vi "ArmControl.vi"   [LabVIEW 2012]
uses:
  Robot Global Data.vi
  State_Machine_Enum.ctl
  <vilib>/Rock Robotics/WPI/Relay/WPI_RelayValue.ctl
types:
  T1 = typedef "State_Machine_Enum.ctl" = enum16{"Idle", "Start", "Do", "Stop", "Init"}
  T2 = typedef "WPI_RelayValue.ctl" = enum16{"Off", "On", "Forward", "Reverse"}
  T3 = typedef "LoopDisable.ctl" = cluster{"Climb.vi":bool, "LauncherAngle.vi":bool, "Launcher.vi":bool, "ArmControl.vi":bool, "WinchMotor.vi":bool, "ReadDriveEncoder.vi":bool}
  T4 = typedef "WPI_RelayDevRef.ctl" = cluster{"DevStatus":errorcluster, "Relay Channel":T5, "Digital Module":T6, "Relay Direction":T7}
  T5 = typedef "FPGA_DIORelayChannel.ctl" = enum8{"Relay 1", "Relay 2", "Relay 3", "Relay 4", "Relay 5", "Relay 6", "Relay 7", "Relay 8", "Invalid"}
  T6 = typedef "FPGA_TypedefDigitalModule.ctl" = enum16{"Digital Module 1", "Digital Module 2"}
  T7 = typedef "WPI_RelayDirection.ctl" = enum16{"Both directions", "Forward only", "Reverse only"}
  T8 = typedef "WPI_DigitalInputDevRef.ctl" = cluster{"DevStatus":errorcluster, "DIO Channel":T9, "Digital Module":T6}
  T9 = typedef "FPGA_DIOChannel.ctl" = enum8{"DIO 1", "DIO 2", "DIO 3", "DIO 4", "DIO 5", "DIO 6", "DIO 7", "DIO 8", "DIO 9", "DIO 10", "DIO 11", "DIO 12", "DIO 13", "DIO 14", "Invalid"}
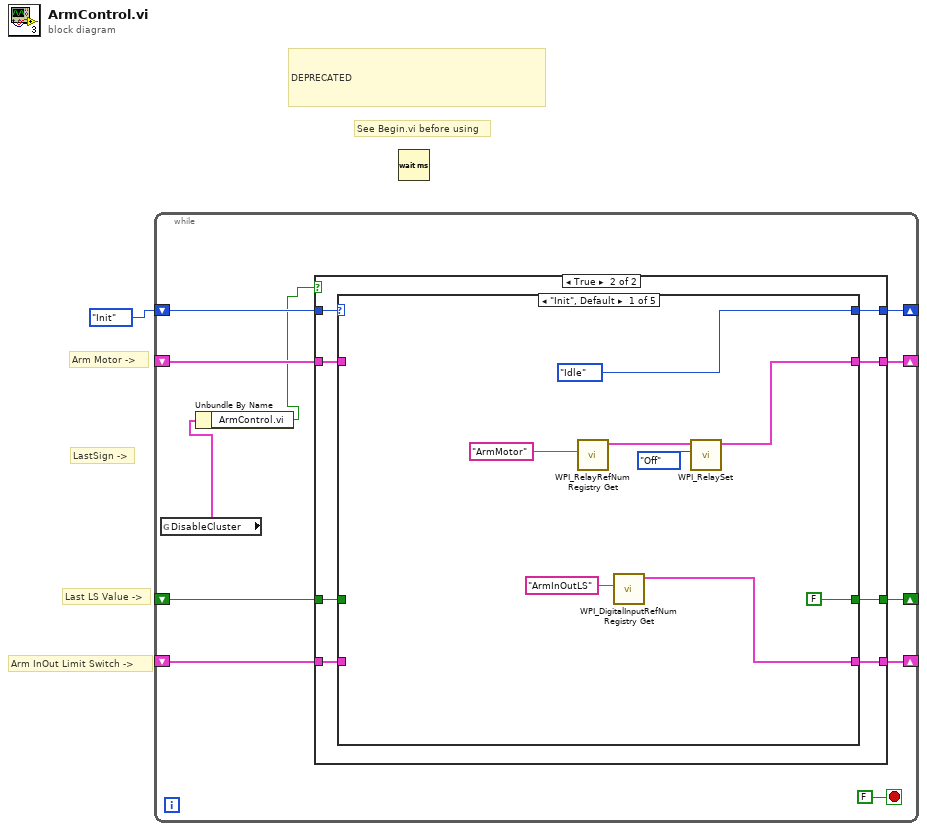
[diagram p0: block diagram]
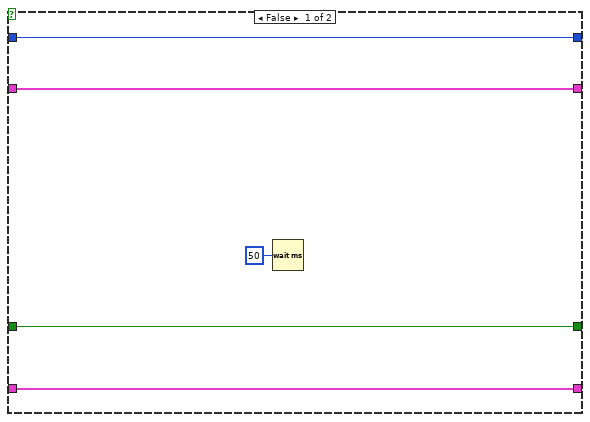
[diagram p2: hidden frame]
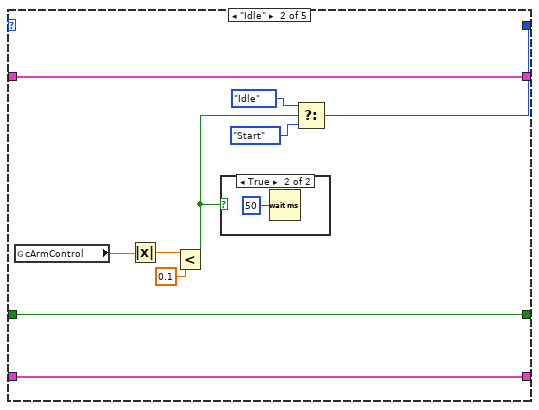
[diagram p3: hidden frame]
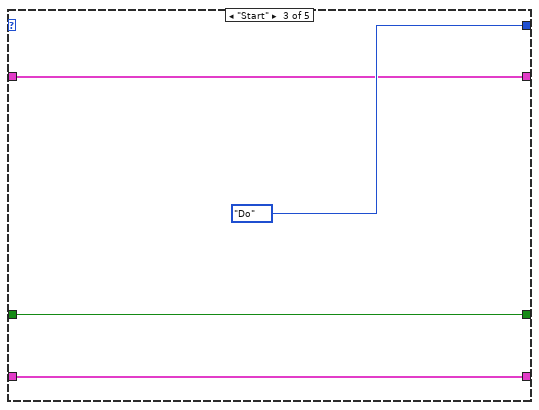
[diagram p5: hidden frame]
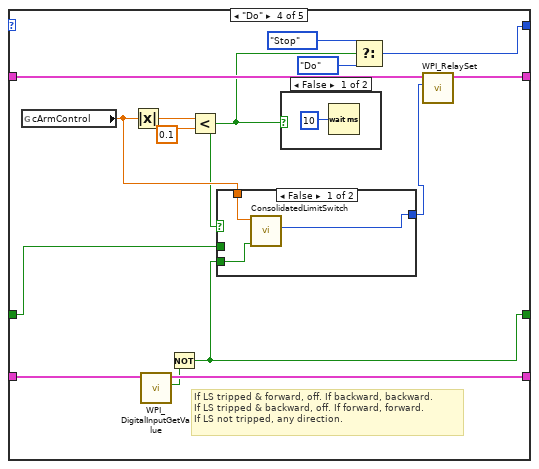
[diagram p6: hidden frame]
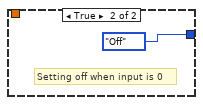
[diagram p7: hidden frame]
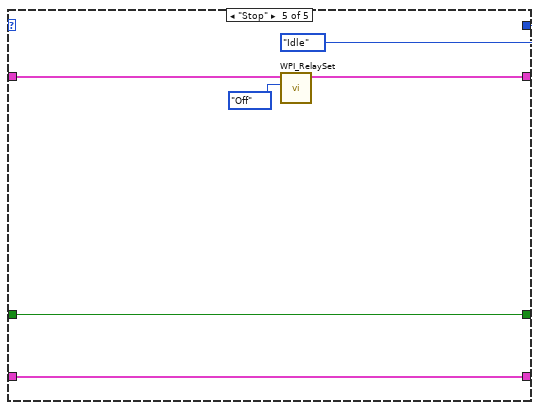
[diagram p9: hidden frame]
diagram:
  # "See Begin.vi before using"
  # "DEPRECATED"
  # "Last LS Value ->"
  # "LastSign ->"
  # "Arm InOut Limit Switch ->"
  # "Arm Motor ->"
  n1 = while {
    shift-right: [w11] -> _
    shift-left: _ -> [w10]
    shift-right: [w8] -> _
    shift-left: State_Machine_Enum."Init" ("State") -> [w9]
    shift-right: [w7] -> _
    shift-left: _ -> [w6]
    shift-right: [w5] -> _
    shift-left: _ -> [w4]
    stop <- FALSE stop-if-true
    n2 = global read "Robot Global Data.vi" "DisableCluster"() -> (w3:T3)
    n3 = Unbundle By Name(w3) -> ("ArmControl.vi"=w2:bool)
    n4 = case shown="True" w2 {
      tunnel: [w15 w25] -> w11
      tunnel: w10 -> [w15 w24]
      tunnel: w9 -> [w13 w23]
      tunnel: [w13 w22] -> w8
      tunnel: [w14 w21] -> w7
      tunnel: w6 -> [w14 w20]
      tunnel: [w16 w19] -> w5
      tunnel: w4 -> [w16 w18]
      frame False {
        n5 = Wait (ms)(milliseconds to wait=u32 50) -> ()  [unwired: 1 out]
      }
      frame True {
        n6 = case shown="\"Init\", Default" w23 {
          tunnel: [w33 w38 w47 w63 w73] -> w25
          tunnel: w24 -> [_ w38 w47 w62 w73]
          tunnel: [State_Machine_Enum."Idle" ("State") w39 State_Machine_Enum."Do" ("f") w57 State_Machine_Enum."Idle" ("State")] -> w22
          tunnel: [w27 w35 w46 w55 w70] -> w21
          tunnel: w20 -> [_ w35 w46 w56 w71]
          tunnel: [FALSE w34 w45 w49 w69] -> w19
          tunnel: w18 -> [_ w34 w45 w52 w69]
          frame "Init", Default {
            n7 = call <vilib>:"WPI_RelayRefNum Registry Get.vi"("refnum name"="ArmMotor") -> ("RelayDevRef"=w29:T4)  [unwired: 9 in, 1 out]
            n8 = call <vilib>:"WPI_DigitalInputRefNum Registry Get.vi"("refnum name"="ArmInOutLS") -> ("DigitalInputDevRef"=w33:T8)  [unwired: 9 in, 1 out]
            n9 = call <vilib>:"WPI_RelaySet.vi"("RelayValue"=WPI_RelayValue."Off", "RelayDevRef"=w29) -> ("RelayDevRef"=w27:T4)  [unwired: 8 in, 1 out]
          }
          frame "Idle" {
            n10 = global read "Robot Global Data.vi" "cArmControl"() -> (w43:dbl)
            n11 = Absolute Value(x=w43) -> (abs(x)=w42:dbl)
            n12 = Less?(x=w42, y=0.1) -> (x < y?=w36:bool)
            n13 = case shown="True" w36 {
              frame False {
              }
              frame True {
                n14 = Wait (ms)(milliseconds to wait=u32 50) -> ()  [unwired: 1 out]
              }
            }
            n15 = Select(t=State_Machine_Enum."Idle" ("f"), s=w36, f=State_Machine_Enum."Start") -> (s? t:f=w39:T1)
          }
          frame "Start" {
          }
          frame "Do" {
            # "If LS tripped & forward, off. If backward, backward.\nIf LS tripped & backward, off. If forward, forward.\nIf LS not tripped, any direction."
            n16 = global read "Robot Global Data.vi" "cArmControl"() -> (w54:dbl)
            n17 = Absolute Value(x=w54) -> (abs(x)=w61:dbl)
            n18 = call <vilib>:"WPI_DigitalInputGetValue.vi"("DigitalInputDevRef"=w62) -> ("Value"=w51:bool, "DigitalInputDevRef"=w63:T8)  [unwired: 8 in, 1 out]
            n19 = Not(x=w51) -> (.not. x?=w49:bool)
            n20 = Less?(x=w61, y=0.1) -> (x < y?=w50:bool)
            n21 = case shown="False" w50 {
              tunnel: w54 -> [w64 _]
              tunnel: [w66 WPI_RelayValue."Off" ("RelayValue")] -> w53
              tunnel: w52 -> [_ _]
              tunnel: w49 -> [w65 _]
              frame False {
                n22 = call "ConsolidatedLimitSwitch.vi"("CurrentLSValue"=w65, "CurrentInput"=w64) -> ("RelayValue"=w66:T2)  [unwired: 9 in]
              }
              frame True {
                # "Setting off when input is 0"
              }
            }
            n23 = case shown="False" w50 {
              frame False {
                n24 = Wait (ms)(milliseconds to wait=u32 10) -> ()  [unwired: 1 out]
              }
              frame True {
              }
            }
            n25 = Select(t=State_Machine_Enum."Stop" ("State"), s=w50, f=State_Machine_Enum."Do" ("State")) -> (s? t:f=w57:T1)
            n26 = call <vilib>:"WPI_RelaySet.vi"("RelayValue"=w53, "RelayDevRef"=w56) -> ("RelayDevRef"=w55:T4)  [unwired: 8 in, 1 out]
          }
          frame "Stop" {
            n27 = call <vilib>:"WPI_RelaySet.vi"("RelayValue"=WPI_RelayValue."Off", "RelayDevRef"=w71) -> ("RelayDevRef"=w70:T4)  [unwired: 8 in, 1 out]
          }
        }
      }
    }
  }
  n28 = Wait (ms)() -> ()  [unwired: 1 in, 1 out]
